vi "VE - Read controller firmware version.vi"(2 "error in":errorcluster, 3 "Address / Port":i16=1 min=1 max=31 step=1) -> (0 "error out":errorcluster, 1 "Read controller \nfirmware version":string)   [LabVIEW 2014]
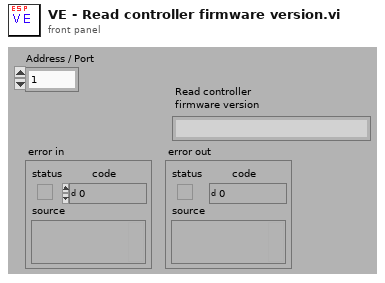
[diagram p1: front panel]
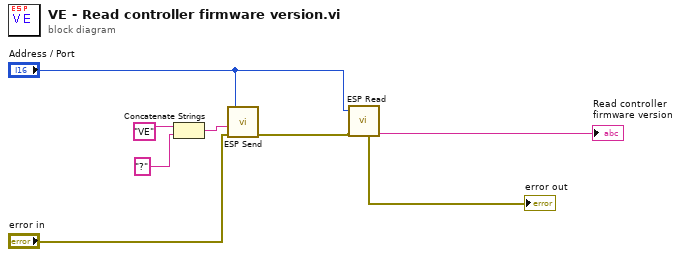
[diagram p0: block diagram]
diagram:
  n1 = Concatenate Strings("VE" ("Substring"), "?" ("Substring")) -> (w7:string)
  n2 = call "ESP Send.vi"("Address / Port"="Address / Port", "Command String"=w7, "error in"="error in") -> ("error out"=w3:errorcluster)  [unwired: 5 in]
  n3 = call "ESP Read.vi"("Address / Port"="Address / Port", "error in"=w3) -> ("error out"=→"error out":errorcluster, "Response String"=→"Read controller \nfirmware version":string)  [unwired: 5 in]
